vi "ActionVIOnCompile.vi"(8 "error in (no error)":errorcluster, 11 "Device Item Ref in":T1 format="%.0x") -> (0 "error out":errorcluster)   [LabVIEW 2018, in "Instrument Addon System Explorer.lvlib"]
uses:
  Instrument Addon System Explorer.lvlib
  <vilib>/NI Veristand/Custom Device API/Custom Device Item Ref.ctl
  Addon Shared/Types/Compiled Settings.ctl
  Addon Shared/Types/Command Parameters.ctl
  Addon Shared/Types/Linked Channel Cluster.ctl
  Addon Shared/Types/Command Channel Indeces.ctl
  Addon Shared/Types/Command Channel Index.ctl
  Addon Shared/Types/Response RT Configuration Cluster.ctl
  Addon Shared/Types/Response Parameters.ctl
  Addon Shared/Types/Response Wait Type.ctl
  Addon Shared/Types/Message Parameters.ctl
  Addon Shared/Types/Message Generation Type.ctl
  Addon Shared/Types/External Trigger Refs.ctl
  <vilib>/NI Veristand/Custom Device API/Data Reference.ctl
  Types/Channel Lookup Cluster.ctl
  Types/Message Channel Lookup Cluster.ctl
  Addon Shared/Types/FG Control.ctl
  Addon Shared/SubVIs/Constants.vi
  <vilib>/NI Veristand/Custom Device Tools/Custom Device Utility Library/NI VeriStand - Search for All Items by GUID.vi
  <vilib>/NI Veristand/Custom Device API/NI VeriStand - Get Item Property.vi
  <vilib>/NI Veristand/Custom Device API/Get Item Property (U32).vi
  <vilib>/NI Veristand/Custom Device API/Get Item Property (Double).vi
  <vilib>/NI Veristand/Custom Device API/Get Item Property (Boolean).vi
  <vilib>/NI Veristand/Custom Device API/Get Item Property (String).vi
  <vilib>/NI Veristand/Custom Device API/Set Item Property (U32).vi
  <vilib>/NI Veristand/Custom Device API/Set Item Property (Double).vi
  <vilib>/NI Veristand/Custom Device API/Set Item Property (Boolean).vi
  <vilib>/NI Veristand/Custom Device API/Set Item Property (String).vi
  <vilib>/NI Veristand/Custom Device Tools/Custom Device Utility Library/NI VeriStand - Get Target Ref.vi
  <vilib>/NI Veristand/Custom Device API/NI VeriStand - Get Channel Data Reference.vi
  <vilib>/NI Veristand/Custom Device Tools/Custom Device Utility Library/NI VeriStand - Get Item Ref by Relative Path.vi
  <vilib>/NI Veristand/Custom Device API/Set Item Property (Variant).vi
  Addon Shared/Instrument Addon Shared.lvlib
  <vilib>/NI Veristand/Custom Device API/Custom Device API.lvlib
  <vilib>/NI Veristand/Custom Device Tools/Custom Device Utility Library/Custom Device Utility Library.lvlib
  <vilib>/NI/NIVS Inline Async API/_Data Access System Explorer/Data Access System Explorer.lvlib
  APIs/Scripting API/Instrument Addon Scripting API.lvlib
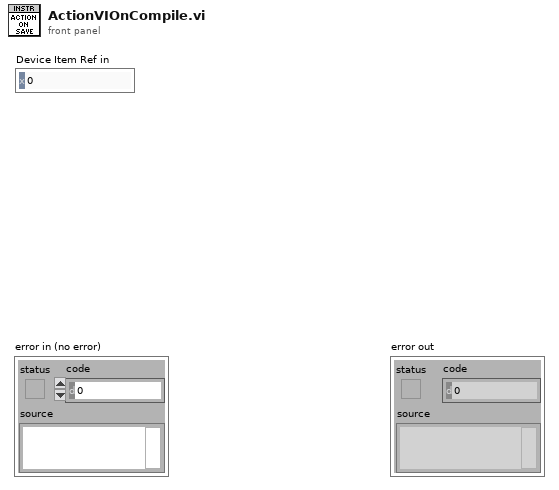
[diagram p1: front panel]
types:
  T1 = typedef "Custom Device API.lvlib/Custom Device Item Ref.ctl" = u64
  T2 = enum16{"Output/Write", "Input/Read", "Input/ReadWrite"}
  T3 = typedef "Instrument Addon System Explorer.lvlib/Message Channel Lookup Cluster.ctl" = cluster{"Status":T1[], "Triggers":T1[], "Periodic Enable":T1[]}
  T4 = typedef "Instrument Addon Shared.lvlib/Compiled Settings.ctl" = cluster{"Command Parameters":T5[], "Command Indeces":T7[], "MetaData Lookup":variant, "Name":string, "Data Lookup":variant, "Response Parameters":T9[], "Message Generation Settings":T12[], "Wait Value Lookup":variant, "Decimation":u32, "External Channels":T14}
  T5 = typedef "Instrument Addon Shared.lvlib/Command Parameters.ctl" = cluster{"Command":string, "Linked Channels":T6[], "Pad":bool, "Length":u32, "Pad Value":u8}
  T6 = typedef "Instrument Addon Shared.lvlib/Linked Channel Cluster.ctl" = cluster{"Variable Name":string, "GUID":string}
  T7 = typedef "Instrument Addon Shared.lvlib/Command Channel Indeces.ctl" = cluster{"Channels":T8[]}
  T8 = typedef "Instrument Addon Shared.lvlib/Command Channel Index.ctl" = cluster{"Data Index":i32, "Data Length":i32}
  T9 = typedef "Instrument Addon Shared.lvlib/Response RT Configuration Cluster.ctl" = cluster{"Reponse Parameters":T10, "Use?":bool}
  T10 = typedef "Instrument Addon Shared.lvlib/Response Parameters.ctl" = cluster{"Response":string, "Linked Channels":T6[], "Type Value":dbl, "Wait Type":T11, "Use Channel":bool, "Channel Path":string}
  T11 = typedef "Instrument Addon Shared.lvlib/Response Wait Type.ctl" = enum16{"Byte Count", "Wait sec"}
  T12 = typedef "Instrument Addon Shared.lvlib/Message Parameters.ctl" = cluster{"Generation Type":T13, "Period":dbl, "Include Protection":bool, "Type":string}
  T13 = typedef "Instrument Addon Shared.lvlib/Message Generation Type.ctl" = enum16{"Trigger Only", "Periodic & Trigger", "Value Change & Trigger"}
  T14 = typedef "Instrument Addon Shared.lvlib/External Trigger Refs.ctl" = cluster{"Channels":T15[], "Triggers":T15[], "Values":dbl[]}
  T15 = typedef "Custom Device API.lvlib/Data Reference.ctl" = i32
  T16 = typedef "Instrument Addon Shared.lvlib/FG Control.ctl" = enum16{"Get", "Set"}
  T17 = cluster{"Name":string, "Type":enum16{"Output/Write", "Input/Read", "Input/ReadWrite"}, "VS Refs":T1[]}
  T18 = typedef "Instrument Addon System Explorer.lvlib/Channel Lookup Cluster.ctl" = cluster{"Lookup":variant, "Index":i32, "Refs":T1[]}
  T19 = typedef "Custom Device API.lvlib/Custom Device Item Info.ctl" = cluster{"Name":string, "Is Channel":bool, "GUID":string, "Is Waveform":bool}
  T20 = typedef "Instrument Addon Shared.lvlib/Trigger Parameters.ctl" = cluster{"Use Channel":bool, "Channel Path":string}
  T21 = cluster{"Name":string, "Type":enum16{"Output/Write", "Input/Read", "Input/ReadWrite"}, "VS Refs":T1[]}[]
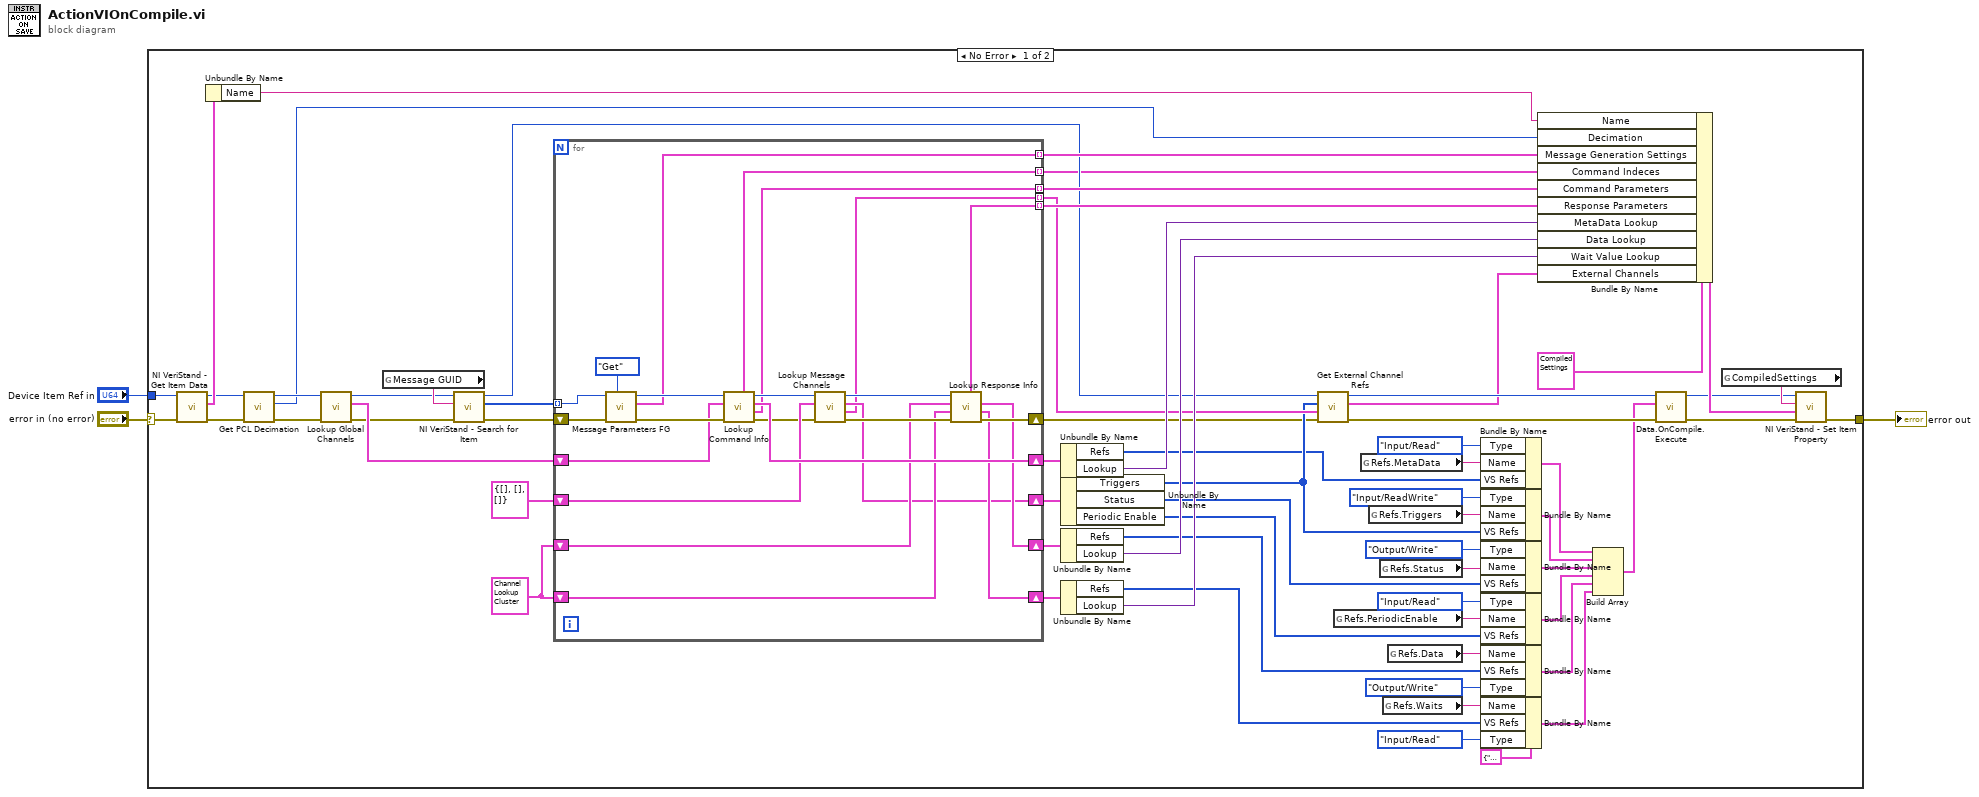
[diagram p0: block diagram]
diagram:
  n1 = case shown="No Error" "error in (no error)" {
    selector: "error in (no error)" -> [w48 w93]
    tunnel: [w47 w93] -> w2
    tunnel: "Device Item Ref in" -> [w49 _]
    frame No Error {
      w17 = T17 {"Name"="", "Type"=enum."Output/Write", "VS Refs"=[]} ("Group")
      w60 = T18 {"Lookup"=variant, "Index"=0, "Refs"=[]} ("Channel Lookup Info")
      n2 = call <vilib>:"NI VeriStand - Get Item Data.vi"("error in (no error)"=w48, "Item Ref in"=w49) -> ("error out"=w8:errorcluster, "Item Info"=w64:T19, "Item Ref out"=w6:T1)  [unwired: 6 in, 1 out]
      n3 = Unbundle By Name(w64) -> ("Name"=w15:string)
      n4 = call "Get PCL Decimation.vi"("Error In"=w8, "Instrument Addon Refnum In"=w6) -> ("Error Out"=w7:errorcluster, "PCL Decimation"=w4:u32, "Instrument Addon Refnum Out"=w5:T1)  [unwired: 7 in]
      n5 = call "Lookup Global Channels.vi"("error in (no error)"=w7, "Item Ref in"=w5) -> ("error out"=w44:errorcluster, "Channel Lookup Info"=w61:T18, "Section Ref out"=w51:T1)  [unwired: 7 in]
      n6 = global read "Constants.vi" "Message GUID"() -> (w69:string)
      n7 = call-poly <vilib>:"NI VeriStand - Search for Item.vi"("error in"=w44, "Item GUID"=w69, "Section Ref in"=w51) -> ("error out"=w67:errorcluster, "Item Refs"=w68:T1[], "Section Ref out"=w36:T1)  [unwired: 5 in, 1 out]
      n8 = for {
        tunnel: w68 -> [w88] mode=indexing
        tunnel: [w74] -> w65 mode=indexing
        shift-right: [w91] -> w37
        shift-left: w67 -> [w90]
        tunnel: [w79] -> w63 mode=indexing
        tunnel: [w73] -> w62 mode=indexing
        shift-right: [w75] -> w54
        shift-left: T3 {"Status"=[], "Triggers"=[], "Periodic Enable"=[]} -> [w77]
        shift-right: [w84] -> w59
        shift-left: w61 -> [w85]
        shift-right: [w82] -> w57
        shift-left: w60 -> [w83]
        shift-right: [w81] -> w53
        shift-left: w60 -> [w80]
        tunnel: [w72] -> w50 mode=indexing
        tunnel: [w70] -> w9 mode=indexing
        n9 = call "Message Parameters FG.vi"("Action"=FG_Control."Get", "error in (no error)"=w90, "Item Ref in"=w88) -> ("error out"=w89:errorcluster, "Message Settings out"=w73:T12, "Item Ref out"=w87:T1)  [unwired: 6 in]
        n10 = call "Lookup Command Info.vi"("error in (no error)"=w89, "Channel Lookup Info in"=w85, "Item Ref in"=w87) -> ("error out"=w71:errorcluster, "Command Parameters"=w74:T5, "Channel Lookup Info out"=w84:T18, "Section Ref out"=w78:T1, "Command Channel Indeces"=w70:T7)  [unwired: 4 in]
        n11 = call "Lookup Message Channels.vi"("error in (no error)"=w71, "Message Channels in"=w77, "Section Ref in"=w78) -> ("error out"=w92:errorcluster, "Trigger Parameters"=w72:T20, "Message Channels out"=w75:T3, "Section Ref out"=w76:T1)  [unwired: 5 in]
        n12 = call "Lookup Response Info.vi"("error in (no error)"=w92, "Wait Value Channel Lookup Info"=w80, "Resp Channel Lookup Info"=w83, "Section Ref in"=w76) -> ("error out"=w91:errorcluster, "Wait Value Channel Lookup Info out"=w81:T18, "Resp Channel Lookup Info out"=w82:T18, "Response Info"=w79:T9)  [unwired: 3 in, 1 out]
      }
      n13 = Unbundle By Name(w59) -> ("Refs"=w14:T1[], "Lookup"=w58:variant)
      n14 = Unbundle By Name(w54) -> ("Triggers"=w38:T1[], "Status"=w13:T1[], "Periodic Enable"=w41:T1[])
      n15 = Unbundle By Name(w57) -> ("Refs"=w12:T1[], "Lookup"=w56:variant)
      n16 = Unbundle By Name(w53) -> ("Refs"=w11:T1[], "Lookup"=w52:variant)
      n17 = call "Get External Channel Refs.vi"("error in (no error)"=w37, "Triggers"=w50, "Internal Trigger Refs"=w38, "Device Ref in"=w36) -> ("error out"=w40:errorcluster, "Refs"=w10:T14, "Item Ref out"=w39:T1)  [unwired: 5 in]
      n18 = global read "Constants.vi" "Refs.PeriodicEnable"() -> (w33:string)
      n19 = global read "Constants.vi" "Refs.MetaData"() -> (w30:string)
      n20 = global read "Constants.vi" "Refs.Triggers"() -> (w31:string)
      n21 = global read "Constants.vi" "Refs.Status"() -> (w32:string)
      n22 = global read "Constants.vi" "Refs.Waits"() -> (w34:string)
      n23 = global read "Constants.vi" "Refs.Data"() -> (w35:string)
      n24 = Bundle By Name(cluster=w17, "Type"=T2."Input/Read", "Name"=w30, "VS Refs"=w14) -> (w23:T17)
      n25 = Bundle By Name(cluster=w17, "Type"=T2."Input/ReadWrite", "Name"=w31, "VS Refs"=w38) -> (w22:T17)
      n26 = Bundle By Name(cluster=w17, "Type"=T2."Output/Write", "Name"=w32, "VS Refs"=w13) -> (w21:T17)
      n27 = Bundle By Name(cluster=w17, "Type"=T2."Input/Read", "Name"=w33, "VS Refs"=w41) -> (w20:T17)
      n28 = Bundle By Name(cluster=w17, "Name"=w35, "VS Refs"=w12, "Type"=T2."Output/Write") -> (w19:T17)
      n29 = Bundle By Name(cluster=w17, "Name"=w34, "VS Refs"=w11, "Type"=T2."Input/Read") -> (w18:T17)
      n30 = Bundle By Name(cluster=T4 {"Command Parameters"=[], "Command Indeces"=[], "MetaData Lookup"=variant, "Name"="", "Data Lookup"=variant, "Response Parameters"=[], "Message Generation Settings"=[], "Wait Value Lookup"=variant, "Decimation"=0, "External Channels"={"Channels"=[], "Triggers"=[], "Values"=[]}} ("Parameters"), "Name"=w15, "Decimation"=w4, "Message Generation Settings"=w62, "Command Indeces"=w9, "Command Parameters"=w65, "Response Parameters"=w63, "MetaData Lookup"=w58, "Data Lookup"=w56, "Wait Value Lookup"=w52, "External Channels"=w10) -> (w46:T4)
      n31 = Build Array(w23, w22, w21, w20, w19, w18) -> (w16:T21)
      n32 = call <vilib>:"Data.OnCompile.Execute.vi"("error in"=w40, "VS Ref Groups"=w16, "Custom Device Ref"=w39) -> ("error out"=w42:errorcluster, "Custom Device Ref"=w43:T1)  [unwired: 7 in]
      n33 = global read "Constants.vi" "CompiledSettings"() -> (w45:string)
      n34 = call-poly <vilib>:"NI VeriStand - Set Item Property.vi"("error in (no error)"=w42, "Value"=w46, "Property Name"=w45, "Item Ref in"=w43) -> ("error out"=w47:errorcluster)  [unwired: 5 in, 2 out]
    }
    frame Error {
    }
  }
  "error out" <- w2
